vi "ErrCheck_Valid Params Name.vi"(8 "Error In":errorcluster, 11 "Macro Command String IN":string="LOOP.Start\t(loop.iterations,3.000);") -> (0 "Error Out":errorcluster, 3 "Invalid Params name?":bool)   [LabVIEW 2012]
doc: "SciScan 1.2 160622"
uses:
  MacroRules_FGV_Commands.ctl
  <vilib>/Utility/error.llb/whitespace.ctl
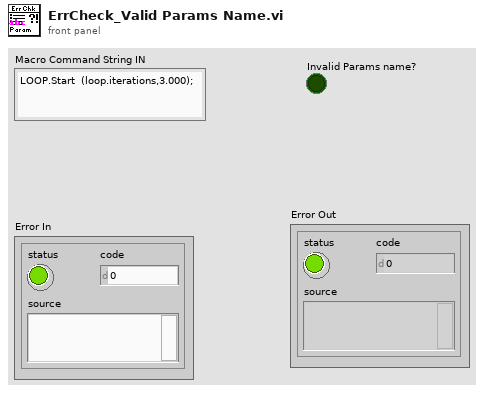
[diagram p1: front panel]
types:
  T1 = typedef "whitespace.ctl" = u16
  T2 = typedef "MacroRules_FGV_Commands.ctl" = enum16{"Read File", "Get All", "Get Param and Flags"}
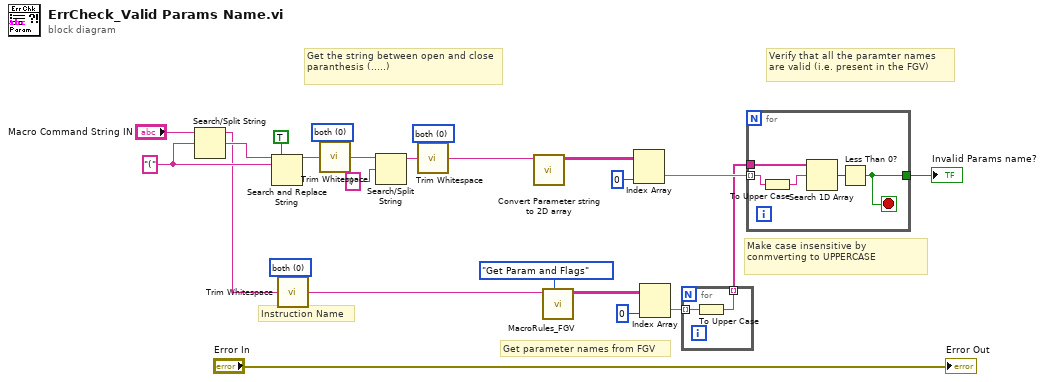
[diagram p0: block diagram]
diagram:
  w5 = T1 0 items=["both", "start of string", "end of string"] ("location (both)")
  w21 = T1 0 items=["both", "start of string", "end of string"] ("location (both)")
  w24 = T1 0 items=["both", "start of string", "end of string"] ("location (both)")
  w10 = "(" ("search string/char (-)")
  # "Make case insensitive by conmverting to UPPERCASE"
  # "Get parameter names from FGV"
  # "Instruction Name"
  # "Verify that all the paramter names are valid (i.e. present in the FGV)"
  # "Get the string between open and close paranthesis (.....)"
  n1 = Search/Split String(string="Macro Command String IN", search string/char (-)=w10) -> (substring before match=w4:string, match + rest of string=w9:string)  [unwired: 1 in, 1 out]
  n2 = Search and Replace String(replace all?=TRUE ("replace all? (F)"), input string=w9, search string=w10) -> (result string=w11:string)  [unwired: 5 in, 3 out]
  n3 = call <vilib>:"Trim Whitespace.vi"("string"=w4, "location (both)"=w5) -> ("trimmed string"=w3:string)
  n4 = call <vilib>:"Trim Whitespace.vi"("string"=w11, "location (both)"=w24) -> ("trimmed string"=w8:string)
  n5 = Search/Split String(string=w8, search string/char (-)=")") -> (substring before match=w22:string)  [unwired: 1 in, 2 out]
  n6 = call <vilib>:"Trim Whitespace.vi"("string"=w22, "location (both)"=w21) -> ("trimmed string"=w6:string)
  n7 = call "Convert Parameter string to 2D array.vi"("Parameter string IN (without paranthesis)"=w6) -> ("Params table OUT"=w16:string[][])  [unwired: 7 in, 3 out]
  n8 = call "MacroRules_FGV.vi"("MacroRules_FGV_Commands"=MacroRules_FGV_Commands."Get Param and Flags", "Command Name IN"=w3) -> ("Parameters"=w7:string[][])  [unwired: 5 in, 4 out]
  n9 = Index Array(array=w16, index (col)=0 ("disabled index (col)")) -> (element=w17:string[])  [unwired: 1 in]
  n10 = Index Array(array=w7, index (col)=0 ("disabled index (col)")) -> (element=w2:string[])  [unwired: 1 in]
  n11 = for {
    tunnel: w2 -> [w26] mode=indexing
    tunnel: [w25] -> w1 mode=indexing
    n12 = To Upper Case(1:w26) -> (0:w25:string)
  }
  n13 = for {
    tunnel: w17 -> [w28] mode=indexing
    tunnel: w1 -> [w31]
    tunnel: [w29] -> w13
    stop <- w29 stop-if-true
    n14 = To Upper Case(1:w28) -> (0:w27:string)
    n15 = Search 1D Array(1D array=w31, element=w27) -> (index of element=w30:i32)  [unwired: 1 in]
    n16 = Less Than 0?(x=w30) -> (x < 0?=w29:bool)
  }
  "Invalid Params name?" <- w13
  "Error Out" <- "Error In"
